vi "Area_Scan_v10 (SubVI).vi"(0 "Step Axis":string, 1 "Scan Termination":T1(ring), 2 "Center of Scan":bool, 3 "Scan Type":enum16{"Sinusoidal", "Spiral"}(ring), 4 "Analog Input":i32, 5 "Table rate":i32, 6 "System no.":i32, 7 "error in (no error)":errorcluster, 8 "Mesh in":dbl, 9 "X-frequency":dbl, 10 "X Scan Range":dbl, 11 "Y-velocity":dbl, 12 "Y Scan Range":dbl, 14 "X Scan Center":dbl, 16 "Y Scan Center":dbl) -> (18 "3D Line Graph":refnum<class "Base Datatype.lvclass">[](array[class]), 20 "Intensity Graph":dbl[][](array[numeric]), 25 "Nano AS Data":dbl[][](array[numeric]), 26 "AS Duration (msec)":u32, 27 "error out":errorcluster)   [LabVIEW 2023]
uses:
  <vilib>/Native 3D Graph/classes/Base Datatype.lvclass
  <vilib>/Native 3D Graph/xcontrol/3DPC_SurfacePlot.xctl
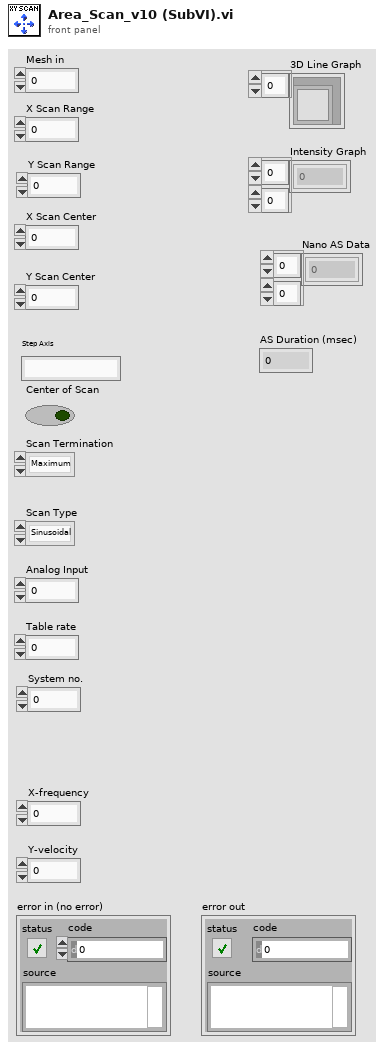
[diagram p1: front panel]
types:
  T1 = enum16{"Maximum", "End Position", "Center of scan", ""}
  T2 = cluster{"Set target type?":bool, "Target type":i32}
  T3 = cluster{"Set stop pos. option?":bool, "Stop pos. option":i32}
  T4 = cluster{"Set centroid method?":bool, "Centroid method":i32}
  T5 = cluster{"Step axis":string, "Range step axis":dbl, "Set Mid. pos?":bool, "Mid. pos. step axis":dbl}
  T6 = cluster{"Scan axis":string, "Range scan axis":dbl, "Set Mid. pos?":bool, "Mid. pos. scan axis":dbl}
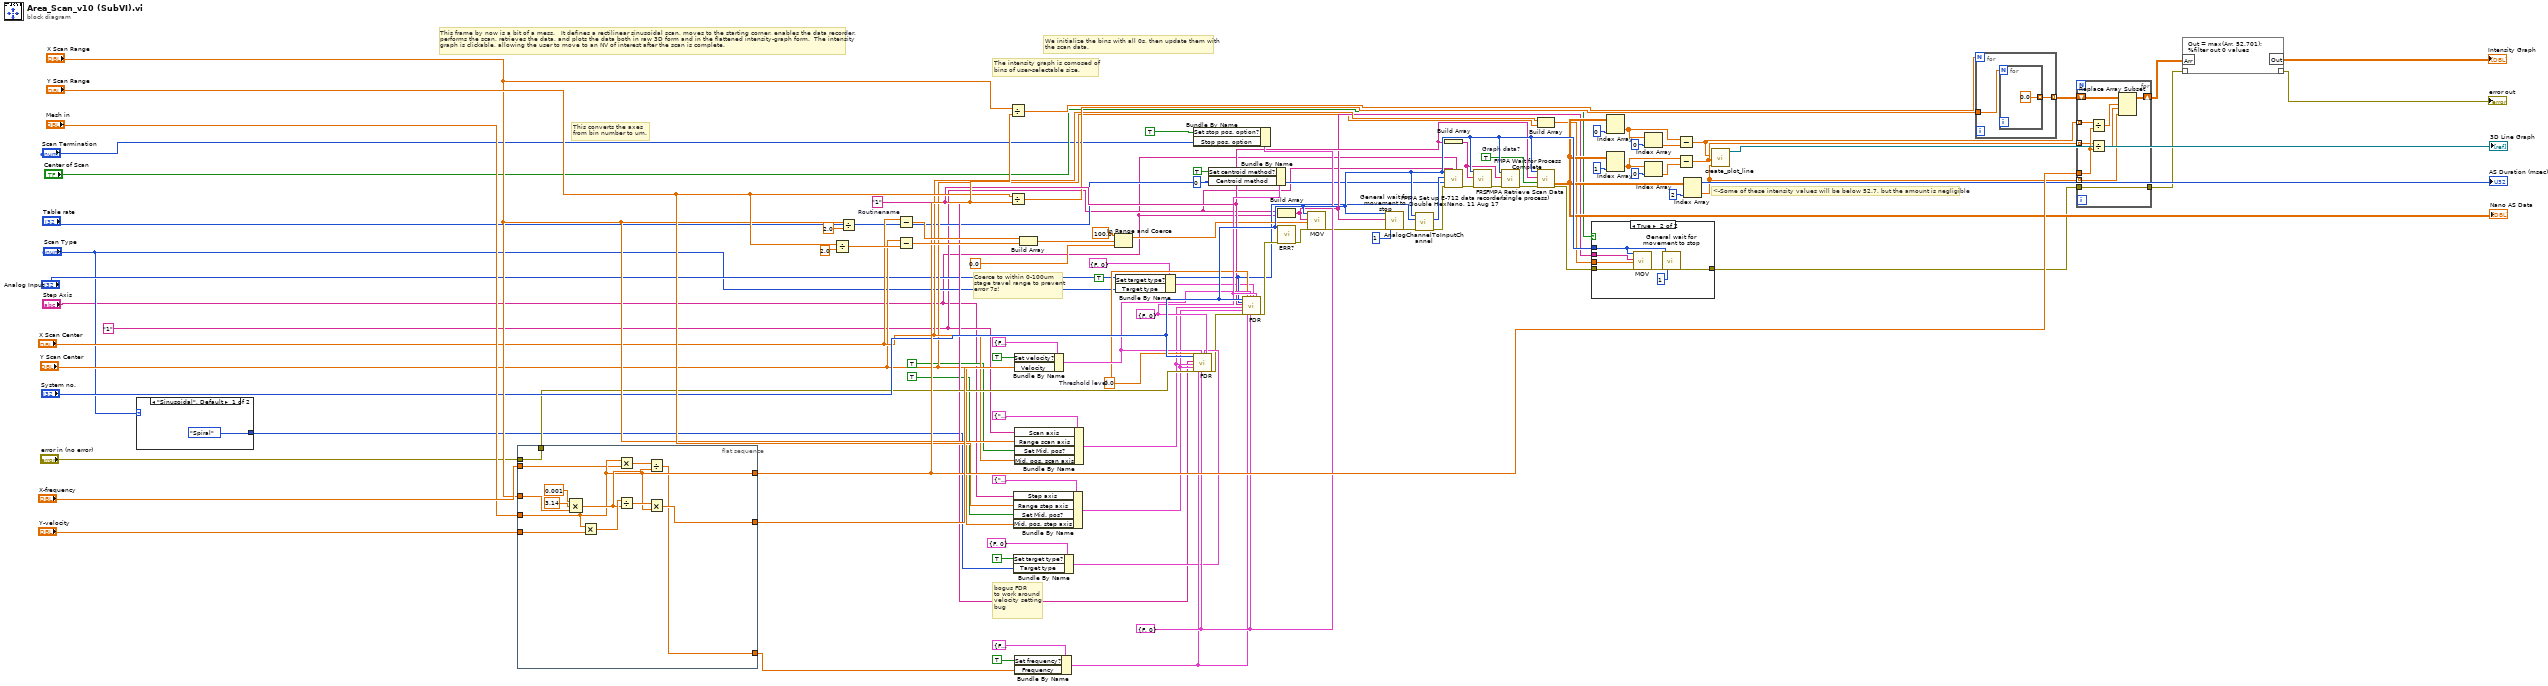
[diagram p0: block diagram]
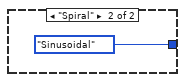
[diagram p2: hidden frame]
diagram:
  w7 = "1"
  w40 = TRUE  # Graph data?
  w79 = T3 {"Set stop pos. option?"=FALSE, "Stop pos. option"=0} ("Stop position option settings")
  w77 = T4 {"Set centroid method?"=FALSE, "Centroid method"=0} ("Centroid method settings")
  w75 = 0.0  # Threshold level
  w69 = "1"  # Routinename
  # "<-Some of these intensity values will be below 52.7, but the amount is negligible"
  # "This converts the axes\nfrom bin number to um."
  # "We initialize the bins with all 0s, then update them with\nthe scan data."
  # "The intensity graph is comosed of\nbins of user-selectable size."
  # "This frame by now is a bit of a mess.   It defines a rectilinear sinusoidal scan, moves to the starting corner, enables the data recorder,\nperforms the scan, retrieves the data, and plots the data both in raw 3D form and in the flattened intensity-graph form.  The intensity\ngraph is clickable, allowing the user to move to an NV of interest after the scan is complete."
  # "bogus FDR\nto work around\nvelocity setting\nbug"
  # "Coerce to within 0-100um\nstage travel range to prevent\nerror 7s!"
  n1 = case shown="\"Sinusoidal\", Default" "Scan Type" {
    tunnel: [enum16{"Sinusoidal", "Spiral"}."Spiral" ("Scan Type") enum16{"Sinusoidal", "Spiral"}."Sinusoidal" ("Scan Type")] -> w11
    frame "Sinusoidal", Default {
    }
    frame "Spiral" {
    }
  }
  n2 = flat-sequence {
    tunnel: "X Scan Range" -> [w107]
    tunnel: [w103] -> w84
    tunnel: "error in (no error)" -> [w103]
    tunnel: "Mesh in" -> [w102]
    tunnel: "X-frequency" -> [w101]
    tunnel: "Y-velocity" -> [w100]
    tunnel: [w102] -> w89
    tunnel: [w99] -> w95
    tunnel: [w98] -> w94
    frame #0 {
      n3 = Compound Arithmetic op=MULTIPLY(0.001, 3.14, w107) -> (w105:dbl)
      n4 = Multiply(x=w102, y=w100) -> (x*y=w106:dbl)
      n5 = Multiply(x=w102, y=w101) -> (x*y=w110:dbl)
      n6 = Divide(x=w106, y=w105) -> (x/y=w104:dbl)
      n7 = Divide(x=w110, y=w105) -> (x/y=w98:dbl)
      n8 = Multiply(x=w104, y=w102) -> (x*y=w99:dbl)
    }
  }
  n9 = Divide(x="Y Scan Range", y=2.0) -> (x/y=w65:dbl)
  n10 = Divide(x="X Scan Range", y=2.0) -> (x/y=w28:dbl)
  n11 = Subtract(x="X Scan Center", y=w28) -> (x-y=w90:dbl)
  n12 = Subtract(x="Y Scan Center", y=w65) -> (x-y=w91:dbl)
  n13 = Divide(x="X Scan Range", y=w89) -> (x/y=w66:dbl)
  n14 = Divide(x="Y Scan Range", y=w89) -> (x/y=w67:dbl)
  n15 = Bundle By Name(cluster=T5 {"Step axis"="", "Range step axis"=0.1, "Set Mid. pos?"=FALSE, "Mid. pos. step axis"=0.1} ("Step axis settings"), "Step axis"="Step Axis", "Range step axis"="Y Scan Range", "Set Mid. pos?"=TRUE, "Mid. pos. step axis"="Y Scan Center") -> (w70:T5)
  n16 = Bundle By Name(cluster=T2 {"Set target type?"=FALSE, "Target type"=0} ("Target type settings"), "Set target type?"=TRUE, "Target type"=w11) -> (w74:T2)
  n17 = Bundle By Name(cluster=cluster{"Set velocity?":bool, "Velocity":dbl} {"Set velocity?"=FALSE, "Velocity"=0.1} ("Velocity settings"), "Set velocity?"=TRUE ("Set target type?"), "Velocity"=w95) -> (w76:cluster{"Set velocity?":bool, "Velocity":dbl})
  n18 = Bundle By Name(cluster=T6 {"Scan axis"="", "Range scan axis"=0.1, "Set Mid. pos?"=FALSE, "Mid. pos. scan axis"=0.1} ("Scan axis settings"), "Scan axis"=w7, "Range scan axis"="X Scan Range", "Set Mid. pos?"=TRUE, "Mid. pos. scan axis"="X Scan Center") -> (w71:T6)
  n19 = Bundle By Name(cluster=cluster{"Set frequency?":bool, "Frequency":dbl} {"Set frequency?"=FALSE, "Frequency"=10.0} ("Frequency settings"), "Set frequency?"=TRUE, "Frequency"=w94) -> (w78:cluster{"Set frequency?":bool, "Frequency":dbl})
  n20 = Build Array(w90, w91) -> (w62:dbl[])
  n21 = In Range and Coerce(upper limit=100.0, x=w62, lower limit=0.0) -> (coerced(x)=w63:dbl[])  [unwired: 1 out]
  n22 = Bundle By Name(cluster=T2 {"Set target type?"=FALSE, "Target type"=0} ("Target type settings"), "Set target type?"=TRUE, "Target type"="Scan Type") -> (w19:T2)
  n23 = Bundle By Name(cluster=w79, "Set stop pos. option?"=TRUE, "Stop pos. option"="Scan Termination") -> ()  [unwired: 1 out]
  n24 = call "FDR.vi"("System no."="System no.", "Routinename"=w69, "Scan axis settings"=w71, "Step axis settings"=w70, "error in"=w84, "Threshold level"=w75, "Frequency settings"=w78, "Velocity settings"=w76, "Stop position option settings"=w79, "Target type settings"=w74, "Centroid method settings"=w77) -> ("error out"=w68:errorcluster)  [unwired: 3 in, 5 out]
  n25 = Bundle By Name(cluster=w77, "Set centroid method?"=TRUE, "Centroid method"=0) -> ()  [unwired: 1 out]
  n26 = call "FDR.vi"("System no."="System no.", "Board"="Analog Input", "Routinename"=w69, "Scan axis settings"=w71, "Step axis settings"=w70, "error in"=w68, "Threshold level"=w75, "Frequency settings"=w78, "Velocity settings"=w76, "Stop position option settings"=w79, "Target type settings"=w19, "Centroid method settings"=w77) -> ("error out"=w47:errorcluster)  [unwired: 2 in, 5 out]
  n27 = Build Array(w7, "Step Axis") -> (w44:string[])
  n28 = call "ERR?.vi"("System no."="System no.", "error in"=w47) -> ("error out"=w48:errorcluster)  [unwired: 16 in, 1 out]
  n29 = call "MOV.vi"("System no."="System no.", "Axes to move"=w44, "Position values"=w63, "error in"=w48) -> ("error out"=w30:errorcluster)  [unwired: 1 in, 14 out]
  n30 = call "General wait for movement to stop.vi"("System no."="System no.", "Axes to wait for"=w44, "error in"=w30, "Polling cycle \ntime, ms"=u32 1 ("Polling cycle \ntime, ms")) -> ("error out"=w31:errorcluster)  [unwired: 4 in, 11 out]
  n31 = call "AnalogChannelToInputChannel.vi"("error in (no error)"=w31, "Optical Channel In"="Analog Input", "System no."="System no.") -> ("error out"=w34:errorcluster, "Input Channel Out"=w41:i32)  [unwired: 7 in]
  n32 = Build Array(w69) -> (w39:string[])
  n33 = call "FMPA Set up E-712 data recorder - Double HexNano, 11 Aug 17.vi"("Step axis sensor ch"="Step Axis", "Scan axis sensor ch"=w7, "error in"=w34, "Table rate"="Table rate", "Opt. Ch."=w41, "System no."="System no.") -> ("error out"=w36:errorcluster)  [unwired: 5 in]
  n34 = call "FRS.vi"("System no."="System no.", "Routines to start"=w39, "error in"=w36) -> ("error out"=w37:errorcluster)  [unwired: 16 in]
  n35 = call "FMPA Wait for Process Complete.vi"("error in"=w37, "Routines to query"=w39, "System no."="System no.") -> ("error out"=w38:errorcluster)  [unwired: 7 in, 1 out]
  n36 = Build Array("X Scan Center", "Y Scan Center") -> (w43:dbl[])
  n37 = call "FMPA Retrieve Scan Data (single process).vi"("System no."="System no.", "Process"=w69, "Graph data?"=w40, "error in"=w38) -> ("Duration (msec)"=→"AS Duration (msec)":u32, "Data"=w58:dbl[][], "error out"=w45:errorcluster)  [unwired: 10 in, 3 out]
  "Nano AS Data" <- w58
  n38 = case shown="True" "Center of Scan" {
    tunnel: w43 -> [_ w116]
    tunnel: w44 -> [_ w115]
    tunnel: w45 -> [w111 w114]
    tunnel: "System no." -> [_ w113]
    tunnel: [w111 w112] -> w12
    frame False {
    }
    frame True {
      n39 = call "MOV.vi"("System no."=w113, "Axes to move"=w115, "Position values"=w116, "error in"=w114) -> ("error out"=w118:errorcluster)  [unwired: 1 in, 14 out]
      n40 = call "General wait for movement to stop.vi"("System no."=w113, "error in"=w118, "Polling cycle \ntime, ms"=u32 1 ("Polling cycle \ntime, ms")) -> ("error out"=w112:errorcluster)  [unwired: 5 in, 11 out]
    }
  }
  n41 = Index Array(array=w58, index (col)=0 ("index")) -> (element=w52:dbl[])  [unwired: 1 in]
  n42 = Index Array(array=w58, index (col)=1 ("index")) -> (element=w49:dbl[])  [unwired: 1 in]
  n43 = Index Array(array=w52, index=0) -> (element=w53:dbl)
  n44 = Index Array(array=w49, index=0) -> (element=w50:dbl)
  n45 = Subtract(x=w52, y=w53) -> (x-y=w81:dbl[])
  n46 = Subtract(x=w49, y=w50) -> (x-y=w82:dbl[])
  n47 = Index Array(array=w58, index (col)=2 ("index")) -> (element=w4:dbl[])  [unwired: 1 in]
  n48 = call <vilib>:"create_plot_line.vi"("z vector"=w4, "y vector"=w82, "x vector"=w81) -> ("plots out"=→"3D Line Graph":refnum<class "Base Datatype.lvclass">[])  [unwired: 2 in, 6 out]
  n49 = for {
    N: w66 -> [_]
    tunnel: [w120] -> w59 mode=indexing
    tunnel: w67 -> [w119]
    n50 = for {
      N: w119 -> [_]
      tunnel: [0.0] -> w120 mode=indexing
    }
  }
  n51 = for {
    tunnel: w4 -> [w126] mode=indexing
    tunnel: w81 -> [w127] mode=indexing
    tunnel: w89 -> [w124]
    shift-right: [w128] -> w5
    shift-left: w59 -> [w125]
    tunnel: w82 -> [w123] mode=indexing
    tunnel: w12 -> [w122]
    tunnel: [w122] -> w2
    n52 = Divide(x=w127, y=w124) -> (x/y=w130:dbl)
    n53 = Divide(x=w123, y=w124) -> (x/y=w129:dbl)
    n54 = Replace Array Subset(array=w125, new element=w126, index (row)=w130, index (col)=w129) -> (w128:dbl[][])
  }
  n55 = script code="Out = max(Arr, 52.701);\n%filter out 0 values"("??"=w2, "Arr"=w5) -> ("??"=→"error out":errorcluster, "Out"=→"Intensity Graph":dbl[][])
